vi "Create Sessions - 1Sess.vi"(6 "initialize and close session behavior":T1, 7 "option string":string, 8 "error in":errorcluster, 9 "reset":bool, 11 "session reservation in":refnum<class "Session Reservation.lvclass">) -> (0 "error out":errorcluster, 1 "channel list":string, 2 "session":refnum<k15>, 3 "session reservation out":refnum<class "Session Reservation.lvclass">)   [LabVIEW 2020, in "MeasurementLink niDCPower.lvlib"]
doc: "Create the NI-DCPower driver session from the <b>session reservation in</b>. Returns an error if more than one NI-DCPower session has been reserved. Use \"Create Sesssion - NSess.vi\" for multiple sessions."
uses:
  MeasurementLink niDCPower.lvlib
  Session Factory/Session Factory.lvclass
  7f77feb2-d2b5-4acd-8f0f-f1b24b7d1641.vi
  MeasurementLink Session Management/Session Reservation/Session Reservation.lvclass
  MeasurementLink Session Management/Session Reservation/Initialize and Close Session Behavior.ctl
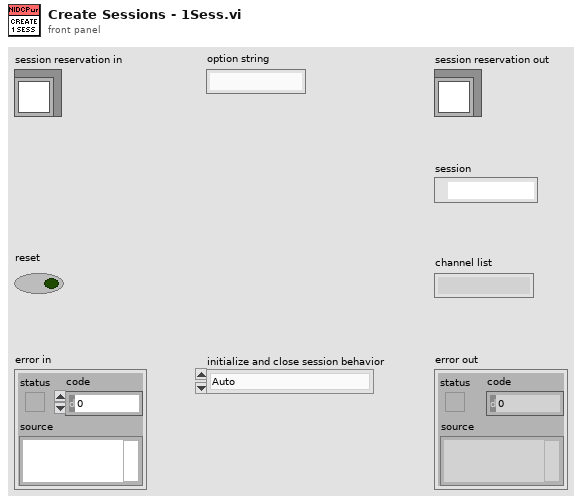
[diagram p1: front panel]
types:
  T1 = typedef "MeasurementLink Session Management.lvlib/Session Reservation.lvclass/Initialize and Close Session Behavior.ctl" = enum16{"Auto", "Initialize and Close", "Attach and Detach", "Initialize and Detach", "Attach and Close"}
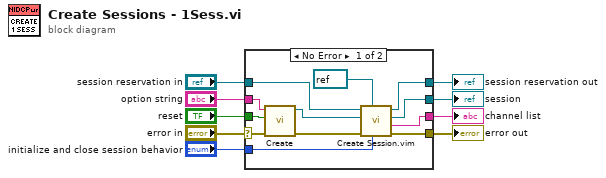
[diagram p0: block diagram]
diagram:
  n1 = case shown="No Error" "error in" {
    selector: "error in" -> [w20 w23]
    tunnel: [w17 w23] -> w8
    tunnel: [w21 w22] -> w6
    tunnel: "session reservation in" -> [w12 w22]
    tunnel: "option string" -> [w18 _]
    tunnel: "reset" -> [w19 _]
    tunnel: [w16 _] -> w3
    tunnel: [w15 _] -> w2
    tunnel: "initialize and close session behavior" -> [w10 _]
    frame No Error {
      n2 = call "Create.vi"("error in"=w20, "reset"=w19, "option string"=w18) -> ("error out"=w11:errorcluster, "instrument out"=w13:refnum<class "Session Factory.lvclass">)  [unwired: 7 in]
      n3 = call "Create Session.vim"("initialize and close session behavior"=w10, "session type"=refnum<k15> refnum ("instrument handle out"), "error in"=w11, "instrument"=w13, "session reservation in"=w12) -> ("error out"=w17:errorcluster, "channel list"=w16:string, "session"=w15:refnum<k15>, "session reservation out"=w21:refnum<class "Session Reservation.lvclass">)  [unwired: 3 in]
    }
    frame Error {
    }
  }
  "error out" <- w8
  "session reservation out" <- w6
  "session" <- w2
  "channel list" <- w3
